vi "measurement_daqmx_task.vi"(8 "error in":errorcluster, 10 "Fast Data Input Physical Channels":T1={"Absolute Pressure"="cDAQ1Mod5/ai20", "Pitot dP"="cDAQ1Mod8/ai8", "PG Temperature 1"="cDAQ1Mod6/ai4", "PG Temperature 2"="cDAQ1Mod6/ai5", "dP Windows 1 to 7"="cDAQ1Mod8/ai11", "dP Windows 1 to 4"="cDAQ1Mod8/ai10", "Camera Voltage"="cDAQ1Mod2/ai0", "dP Windows 1 to 4 F"="cDAQ1Mod2/ai0", "TS Temperature 1"="cDAQ1Mod2/ai0", "TS Temperature 2"="cDAQ1Mod2/ai0", "TS Abs Pressure 1"="cDAQ1Mod2/ai0", "TS Abs Pressure 2"="cDAQ1Mod2/ai0", "Main Diode"="cDAQ1Mod2/ai0", "Temperature Diode"="cDAQ1Mod2/ai0", "TS Exterior Temp"="cDAQ1Mod2/ai0", "DS Exterior Temp"="cDAQ1Mod2/ai0", "Vapor Line Pitot dP"="cDAQ1Mod3/ai6"}, 11 "task in":refnum<k21>) -> (0 "error out":errorcluster, 3 "task out":refnum<k21>)   [LabVIEW 2017]
uses:
  Input Channel Lists/pulse_generator_input_physical_channels.ctl
  <vilib>/DAQmx/create/channels.llb/DAQmx Create Channel (AI-Voltage-Basic).vi
  <vilib>/DAQmx/create/channels.llb/DAQmx Create Channel (AI-Current-Basic).vi
  <vilib>/DAQmx/create/channels.llb/DAQmx Create Channel (AI-Temperature-Thermocouple).vi
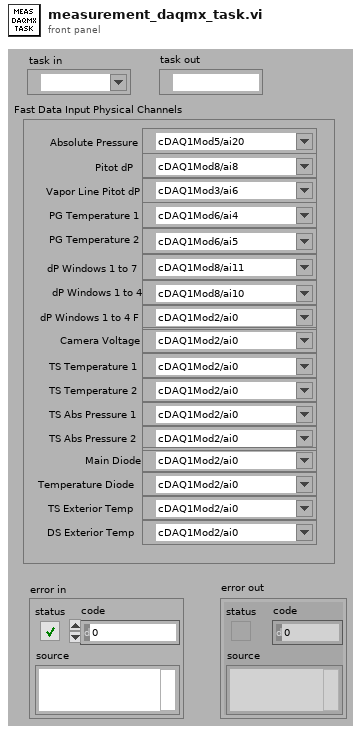
[diagram p1: front panel]
types:
  T1 = typedef "pulse_generator_input_physical_channels.ctl" = cluster{"Absolute Pressure":tag, "Pitot dP":tag, "PG Temperature 1":tag, "PG Temperature 2":tag, "dP Windows 1 to 7":tag, "dP Windows 1 to 4":tag, "Camera Voltage":tag, "dP Windows 1 to 4 F":tag, "TS Temperature 1":tag, "TS Temperature 2":tag, "TS Abs Pressure 1":tag, "TS Abs Pressure 2":tag, "Main Diode":tag, "Temperature Diode":tag, "TS Exterior Temp":tag, "DS Exterior Temp":tag, "Vapor Line Pitot dP":tag}
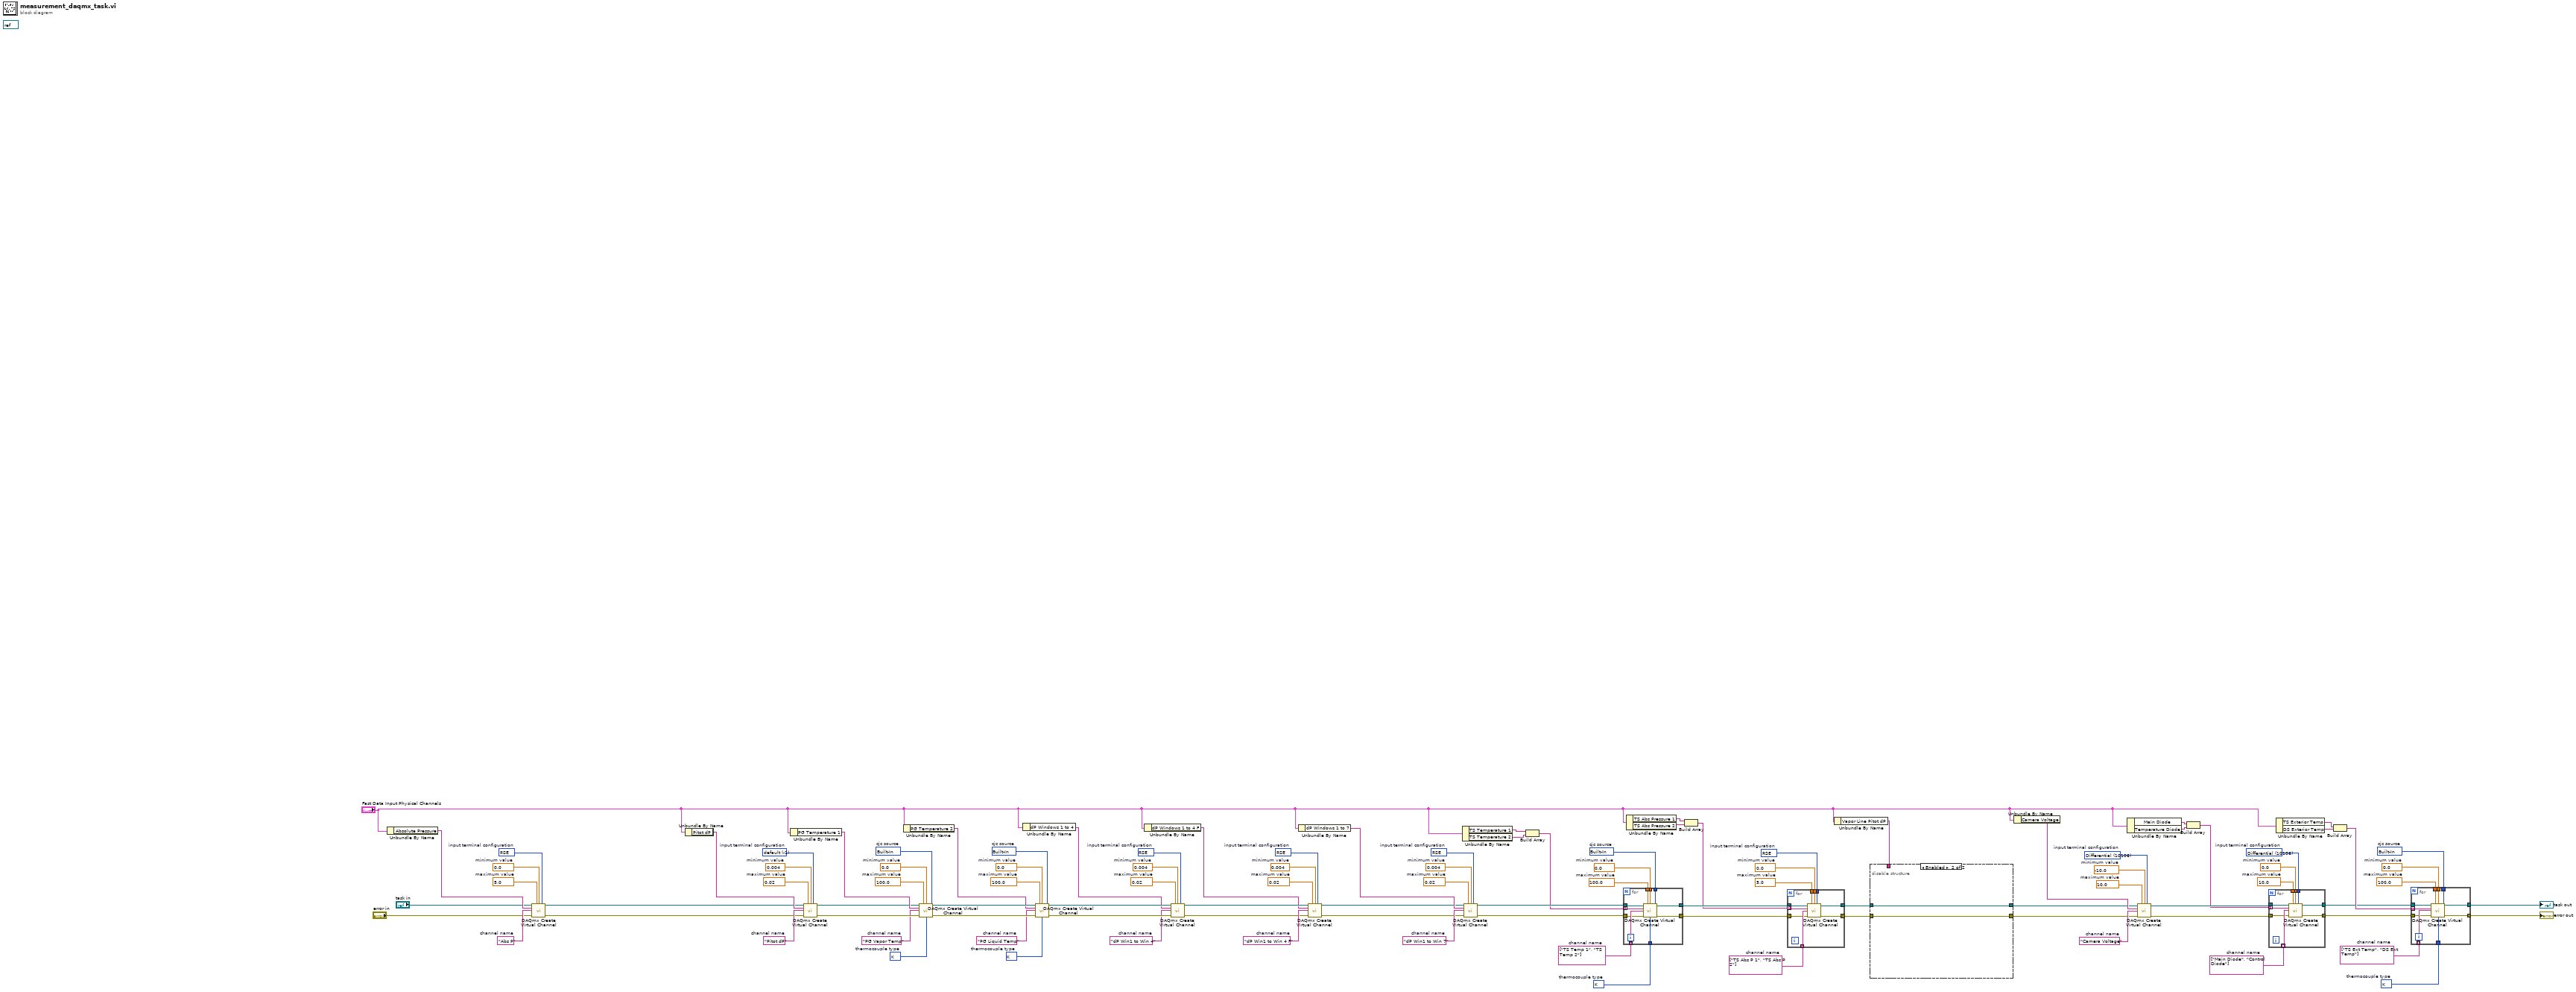
[diagram p0: block diagram]
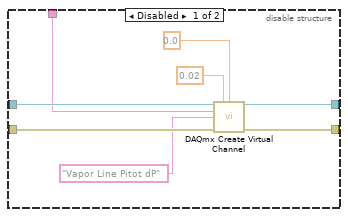
[diagram p2: hidden frame]
diagram:
  w17 = 10106 items=["default"=-1, "RSE"=10083, "NRSE"=10078, "Differential"=10106, "Pseudodifferential"=12529]  # input terminal configuration
  w18 = string[] ["Main Diode", "Control Diode"]  # channel name
  w19 = 0.0  # minimum value
  w20 = 10.0  # maximum value
  w24 = 10200 items=["Built-In"=10200, "Constant Value"=10116, "Channel"=10113]  # cjc source
  w26 = 10073 items=["J"=10072, "K"=10073, "N"=10077, "R"=10082, "S"=10085, "T"=10086, "B"=10047, "E"=10055]  # thermocouple type
  w25 = string[] ["TS Ext Temp", "DS Ext Temp"]  # channel name
  w27 = 0.0  # minimum value
  w28 = 100.0  # maximum value
  w38 = 10083 items=["default"=-1, "RSE"=10083, "NRSE"=10078, "Differential"=10106, "Pseudodifferential"=12529]  # input terminal configuration
  w37 = "dP Win1 to Win 4 F"  # channel name
  w36 = 0.004  # minimum value
  w35 = 0.02  # maximum value
  w51 = 10083 items=["default"=-1, "RSE"=10083, "NRSE"=10078, "Differential"=10106, "Pseudodifferential"=12529]  # input terminal configuration
  w50 = string[] ["TS Abs P 1", "TS Abs P 2"]  # channel name
  w49 = 0.0  # minimum value
  w48 = 5.0  # maximum value
  w58 = 10200 items=["Built-In"=10200, "Constant Value"=10116, "Channel"=10113]  # cjc source
  w56 = 10073 items=["J"=10072, "K"=10073, "N"=10077, "R"=10082, "S"=10085, "T"=10086, "B"=10047, "E"=10055]  # thermocouple type
  w57 = string[] ["TS Temp 1", "TS Temp 2"]  # channel name
  w55 = 0.0  # minimum value
  w54 = 100.0  # maximum value
  (unwired) refnum<k21> refnum ("task out")
  w68 = 10106 items=["default"=-1, "RSE"=10083, "NRSE"=10078, "Differential"=10106, "Pseudodifferential"=12529]  # input terminal configuration
  w69 = "Camera Voltage"  # channel name
  w70 = -10.0  # minimum value
  w71 = 10.0  # maximum value
  w72 = 10083 items=["default"=-1, "RSE"=10083, "NRSE"=10078, "Differential"=10106, "Pseudodifferential"=12529]  # input terminal configuration
  w73 = "dP Win1 to Win 7"  # channel name
  w74 = 0.004  # minimum value
  w75 = 0.02  # maximum value
  w76 = 10083 items=["default"=-1, "RSE"=10083, "NRSE"=10078, "Differential"=10106, "Pseudodifferential"=12529]  # input terminal configuration
  w77 = "dP Win1 to Win 4"  # channel name
  w78 = 0.004  # minimum value
  w79 = 0.02  # maximum value
  w81 = 10200 items=["Built-In"=10200, "Constant Value"=10116, "Channel"=10113]  # cjc source
  w83 = 10073 items=["J"=10072, "K"=10073, "N"=10077, "R"=10082, "S"=10085, "T"=10086, "B"=10047, "E"=10055]  # thermocouple type
  w82 = "PG Liquid Temp"  # channel name
  w85 = 0.0  # minimum value
  w86 = 100.0  # maximum value
  w88 = 10200 items=["Built-In"=10200, "Constant Value"=10116, "Channel"=10113]  # cjc source
  w90 = 10073 items=["J"=10072, "K"=10073, "N"=10077, "R"=10082, "S"=10085, "T"=10086, "B"=10047, "E"=10055]  # thermocouple type
  w89 = "PG Vapor Temp"  # channel name
  w92 = 0.0  # minimum value
  w93 = 100.0  # maximum value
  w94 = -1 items=["default"=-1, "RSE"=10083, "NRSE"=10078, "Differential"=10106, "Pseudodifferential"=12529]  # input terminal configuration
  w95 = "Pitot dP"  # channel name
  w97 = 0.004  # minimum value
  w98 = 0.02  # maximum value
  w99 = 10083 items=["default"=-1, "RSE"=10083, "NRSE"=10078, "Differential"=10106, "Pseudodifferential"=12529]  # input terminal configuration
  w100 = "Abs P"  # channel name
  w101 = 0.0  # minimum value
  w102 = 5.0  # maximum value
  n1 = Unbundle By Name("Fast Data Input Physical Channels") -> ("Absolute Pressure"=w67:tag)
  n2 = call-poly <vilib>:"DAQmx Create Virtual Channel.vi"("task in"="task in", "maximum value"=w102, "minimum value"=w101, "input terminal configuration"=w99, "physical channels"=w67, "name to assign"=w100, "error in"="error in") -> ("task out"=w40:refnum<k21>, "error out"=w39:errorcluster)  [unwired: 7 in]
  n3 = Unbundle By Name("Fast Data Input Physical Channels") -> ("Pitot dP"=w66:tag)
  n4 = Unbundle By Name("Fast Data Input Physical Channels") -> ("PG Temperature 1"=w65:tag)
  n5 = call-poly <vilib>:"DAQmx Create Virtual Channel.vi"("task in"=w40, "maximum value"=w98, "minimum value"=w97, "input terminal configuration"=w94, "physical channels"=w66, "name to assign"=w95, "error in"=w39) -> ("task out"=w7:refnum<k21>, "error out"=w96:errorcluster)  [unwired: 7 in]
  n6 = Unbundle By Name("Fast Data Input Physical Channels") -> ("PG Temperature 2"=w64:tag)
  n7 = call-poly <vilib>:"DAQmx Create Virtual Channel.vi"("task in"=w7, "maximum value"=w93, "minimum value"=w92, "physical channels"=w65, "cjc source"=w88, "name to assign"=w89, "error in"=w96, "thermocouple type"=w90) -> ("task out"=w87:refnum<k21>, "error out"=w91:errorcluster)  [unwired: 6 in]
  n8 = Unbundle By Name("Fast Data Input Physical Channels") -> ("dP Windows 1 to 4"=w63:tag)
  n9 = call-poly <vilib>:"DAQmx Create Virtual Channel.vi"("task in"=w87, "maximum value"=w86, "minimum value"=w85, "physical channels"=w64, "cjc source"=w81, "name to assign"=w82, "error in"=w91, "thermocouple type"=w83) -> ("task out"=w80:refnum<k21>, "error out"=w84:errorcluster)  [unwired: 6 in]
  n10 = Unbundle By Name("Fast Data Input Physical Channels") -> ("dP Windows 1 to 4 F"=w30:tag)
  n11 = call-poly <vilib>:"DAQmx Create Virtual Channel.vi"("task in"=w80, "maximum value"=w79, "minimum value"=w78, "input terminal configuration"=w76, "physical channels"=w63, "name to assign"=w77, "error in"=w84) -> ("task out"=w34:refnum<k21>, "error out"=w33:errorcluster)  [unwired: 7 in]
  n12 = Unbundle By Name("Fast Data Input Physical Channels") -> ("dP Windows 1 to 7"=w62:tag)
  n13 = call-poly <vilib>:"DAQmx Create Virtual Channel.vi"("task in"=w34, "maximum value"=w35, "minimum value"=w36, "input terminal configuration"=w38, "physical channels"=w30, "name to assign"=w37, "error in"=w33) -> ("task out"=w32:refnum<k21>, "error out"=w31:errorcluster)  [unwired: 7 in]
  n14 = Unbundle By Name("Fast Data Input Physical Channels") -> ("TS Temperature 1"=w45:tag, "TS Temperature 2"=w44:tag)
  n15 = call-poly <vilib>:"DAQmx Create Virtual Channel.vi"("task in"=w32, "maximum value"=w75, "minimum value"=w74, "input terminal configuration"=w72, "physical channels"=w62, "name to assign"=w73, "error in"=w31) -> ("task out"=w53:refnum<k21>, "error out"=w52:errorcluster)  [unwired: 7 in]
  n16 = Build Array(w45, w44) -> (w43:tag[])
  n17 = for {
    tunnel: w58 -> [w112]
    tunnel: w57 -> [w111] mode=indexing
    tunnel: w56 -> [w110]
    tunnel: w55 -> [w109]
    tunnel: w54 -> [w108]
    tunnel: w53 -> [w107]
    tunnel: [w105] -> w47
    tunnel: w52 -> [w106]
    tunnel: [w104] -> w46
    tunnel: w43 -> [w103] mode=indexing
    n18 = call-poly <vilib>:"DAQmx Create Virtual Channel.vi"("task in"=w107, "maximum value"=w108, "minimum value"=w109, "physical channels"=w103, "cjc source"=w112, "name to assign"=w111, "error in"=w106, "thermocouple type"=w110) -> ("task out"=w105:refnum<k21>, "error out"=w104:errorcluster)  [unwired: 6 in]
  }
  n19 = Unbundle By Name("Fast Data Input Physical Channels") -> ("TS Abs Pressure 1"=w42:tag, "TS Abs Pressure 2"=w29:tag)
  n20 = Build Array(w42, w29) -> (w41:tag[])
  n21 = for {
    tunnel: w51 -> [w121]
    tunnel: w50 -> [w120] mode=indexing
    tunnel: w49 -> [w119]
    tunnel: w48 -> [w118]
    tunnel: w47 -> [w117]
    tunnel: [w115] -> w6
    tunnel: w46 -> [w116]
    tunnel: [w114] -> w5
    tunnel: w41 -> [w113] mode=indexing
    n22 = call-poly <vilib>:"DAQmx Create Virtual Channel.vi"("task in"=w117, "maximum value"=w118, "minimum value"=w119, "input terminal configuration"=w121, "physical channels"=w113, "name to assign"=w120, "error in"=w116) -> ("task out"=w115:refnum<k21>, "error out"=w114:errorcluster)  [unwired: 7 in]
  }
  n23 = Unbundle By Name("Fast Data Input Physical Channels") -> ("Vapor Line Pitot dP"=w1:tag)
  n24 = disable-structure shown="Enabled" {
    disable-tunnel: w6 -> [w129 w131]
    disable-tunnel: w5 -> [w128 w130]
    disable-tunnel: [w127 w131] -> w4
    disable-tunnel: [w126 w130] -> w3
    disable-tunnel: w1 -> [w125 _]
    frame Disabled {
      n25 = call-poly <vilib>:"DAQmx Create Virtual Channel.vi"("task in"=w129, "maximum value"=0.02, "minimum value"=0.0, "physical channels"=w125, "name to assign"="Vapor Line Pitot dP", "error in"=w128) -> ("task out"=w127:refnum<k21>, "error out"=w126:errorcluster)  [unwired: 8 in]
    }
    frame Enabled {
    }
  }
  n26 = Unbundle By Name("Fast Data Input Physical Channels") -> ("Camera Voltage"=w61:tag)
  n27 = Unbundle By Name("Fast Data Input Physical Channels") -> ("Main Diode"=w14:tag, "Temperature Diode"=w13:tag)
  n28 = call-poly <vilib>:"DAQmx Create Virtual Channel.vi"("task in"=w4, "maximum value"=w71, "minimum value"=w70, "input terminal configuration"=w68, "physical channels"=w61, "name to assign"=w69, "error in"=w3) -> ("task out"=w16:refnum<k21>, "error out"=w15:errorcluster)  [unwired: 7 in]
  n29 = Build Array(w14, w13) -> (w12:tag[])
  n30 = for {
    tunnel: w17 -> [w140]
    tunnel: w18 -> [w139] mode=indexing
    tunnel: w19 -> [w138]
    tunnel: w20 -> [w137]
    tunnel: w16 -> [w136]
    tunnel: [w134] -> w11
    tunnel: w15 -> [w135]
    tunnel: [w133] -> w10
    tunnel: w12 -> [w132] mode=indexing
    n31 = call-poly <vilib>:"DAQmx Create Virtual Channel.vi"("task in"=w136, "maximum value"=w137, "minimum value"=w138, "input terminal configuration"=w140, "physical channels"=w132, "name to assign"=w139, "error in"=w135) -> ("task out"=w134:refnum<k21>, "error out"=w133:errorcluster)  [unwired: 7 in]
  }
  n32 = Unbundle By Name("Fast Data Input Physical Channels") -> ("TS Exterior Temp"=w22:tag, "DS Exterior Temp"=w23:tag)
  n33 = Build Array(w22, w23) -> (w21:tag[])
  n34 = for {
    tunnel: w24 -> [w150]
    tunnel: w25 -> [w149] mode=indexing
    tunnel: w26 -> [w148]
    tunnel: w27 -> [w147]
    tunnel: w28 -> [w146]
    tunnel: [w144] -> w9
    tunnel: w10 -> [w145]
    tunnel: [w143] -> w8
    tunnel: w11 -> [w142]
    tunnel: w21 -> [w141] mode=indexing
    n35 = call-poly <vilib>:"DAQmx Create Virtual Channel.vi"("task in"=w142, "maximum value"=w146, "minimum value"=w147, "physical channels"=w141, "cjc source"=w150, "name to assign"=w149, "error in"=w145, "thermocouple type"=w148) -> ("task out"=w144:refnum<k21>, "error out"=w143:errorcluster)  [unwired: 6 in]
  }
  "error out" <- w8
  "task out" <- w9
